vi "_FPGA Wait Done.vi"(4 "error in":errorcluster, 5 "Timeout (2000ms)":u32=2000, 6 "Indicator":T1) -> (0 "error out":errorcluster)   [LabVIEW 2012]
uses:
  Type/_FPGA Indicator.ctl
  Type/_RW Status.ctl
  _RT Global.vi
  <vilib>/Utility/error.llb/Error Cluster From Error Code.vi
  <vilib>/rvi/errors/niLvFpgaAdjustHostInterfaceError.vi
  <vilib>/rvi/interface/nirviReadWriteControl/nirviReadWriteControl.xnode
  FPGA Bitfiles/FPGA9606.lvbitx
  NiFpgaLv.dll
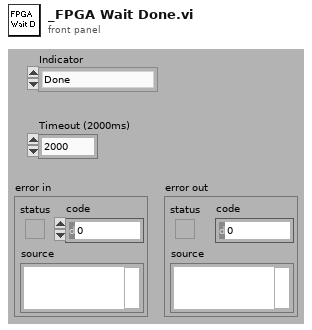
[diagram p1: front panel]
types:
  T1 = typedef "_FPGA Indicator.ctl" = enum16{"Done", "Ready", "Count Available", "SendSerial", "LED State"}
  T2 = typedef "_RW Status.ctl" = enum8{"Done", "Do Read", "Do Write", "Set Latch1", "Set Latch2", "Set Latch3", "Set Latch4", "RP ON", "EL ON", "Serial Send", "Set LC Out", "Get LC In", "Read VAC", "Table Test", "Get Interlock", "Do Read2", "Do Write2"}
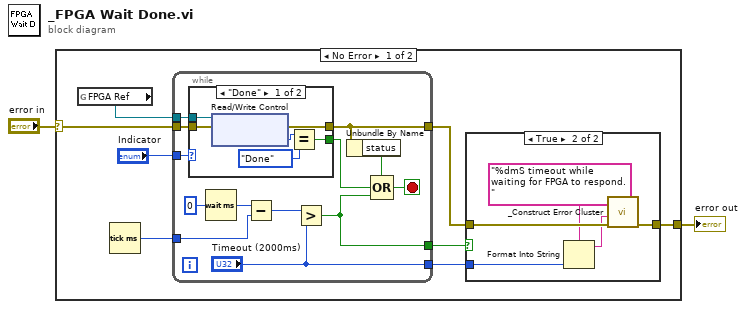
[diagram p0: block diagram]
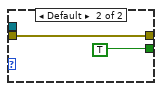
[diagram p3: hidden frame]
diagram:
  n1 = case shown="No Error" "error in" {
    selector: "error in" -> [w5 w38]
    tunnel: [w7 w38] -> w2
    frame No Error {
      n2 = global read "_RT Global.vi" "FPGA Ref"() -> (w3:refnum<k20>)
      n3 = Tick Count (ms)() -> (millisecond timer value=w10:u32)
      n4 = while {
        tunnel: w3 -> [w29]
        tunnel: w5 -> [w28]
        tunnel: [w20] -> w8
        tunnel: w10 -> [w27]
        tunnel: [w23] -> w9
        tunnel: "Indicator" -> [w22]
        tunnel: ["Timeout (2000ms)"] -> w4
        stop <- w24 stop-if-true
        n5 = case shown="\"Done\"" w22 {
          tunnel: w29 -> [w35 _]
          tunnel: w28 -> [w34 w37]
          tunnel: [w33 w37] -> w20
          tunnel: [w32 TRUE] -> w25
          frame "Done" {
            n6 = xnode "Read/Write Control"("FPGA VI Reference In"=w35, "error in"=w34) -> ("error out"=w33:errorcluster, "R/W Status"=w31:T2)  [unwired: 1 out]
            n7 = Equal?(x=w31, y=_RW_Status."Done" ("R/W Status")) -> (x = y?=w32:bool)
          }
          frame Default {
          }
        }
        n8 = Wait (ms)(milliseconds to wait=u32 0) -> (millisecond timer value=w18:u32)
        n9 = Subtract(x=w18, y=w27) -> (x-y=w26:u32)
        n10 = Greater?(x=w26, y="Timeout (2000ms)") -> (0:w23:bool)
        n11 = Unbundle By Name(w20) -> ("status"=w19:bool)
        n12 = Compound Arithmetic op=OR(w19, w25, w23) -> (w24:bool)
      }
      n13 = case shown="True" w9 {
        tunnel: w8 -> [w11 w16]
        tunnel: [w11 w15] -> w7
        tunnel: w4 -> [_ w12]
        frame False {
        }
        frame True {
          n14 = Format Into String(format string="%dmS timeout while waiting for FPGA to respond.", w12) -> (resulting string=w13:string)  [unwired: 2 in, 1 out]
          n15 = call "_Construct Error Cluster.vi"("error in"=w16, "reason"=w13) -> ("error out"=w15:errorcluster)  [unwired: 2 in, 3 out]
        }
      }
    }
    frame Error {
    }
  }
  "error out" <- w2
